vi "Temperature sensors calibration.vi"() -> ()   [LabVIEW 2021]
uses:
  <instrlib>/Lake Shore 350/Public/Data/Sensor Data (Single Reading).vi
  <vilib>/Utility/file.llb/Write Delimited Spreadsheet (DBL).vi
  <instrlib>/Keithley 2450/Keithley 2450.lvlib
  <instrlib>/Lake Shore 350/Lake Shore 350.lvlib
panel:
  out "Chart":T1(graph)
  out "Channel C (Ohm)":dbl format="%#.5f"
  out "Channel B (K)":dbl format="%#.5f"
  out "Channel B (Ohm)":dbl format="%#.5f"
  out "error out write file":errorcluster
  in  "SM1":string
  in  "SM2":string
  out "All data":dbl[][](array[numeric])
  out "SM2 (Omh)":dbl
  in  "error in (no error) 2":errorcluster
  in  "Keithley 2":refnum<visa-resource-name>
  out "VTI Temperature (K)":dbl format="%#.5f"
  out "Waveform Chart":cluster{"Sensor Data":dbl, "Sensor Data":dbl}(graph)
  out "error out":errorcluster
  out "XY Graph":cluster{dbl[], dbl[]}[](graph)
  out "Channel D (Ohm)":dbl format="%#.5f"
  in  "LakeShore 350":refnum<visa-resource-name>="COM4"
  in  "start":bool
  in  "milliseconds to wait":u32=2000
  in  "error in (no error)":errorcluster
  out "SM1 (Omh)":dbl
  in  "Keithley 1":refnum<visa-resource-name>
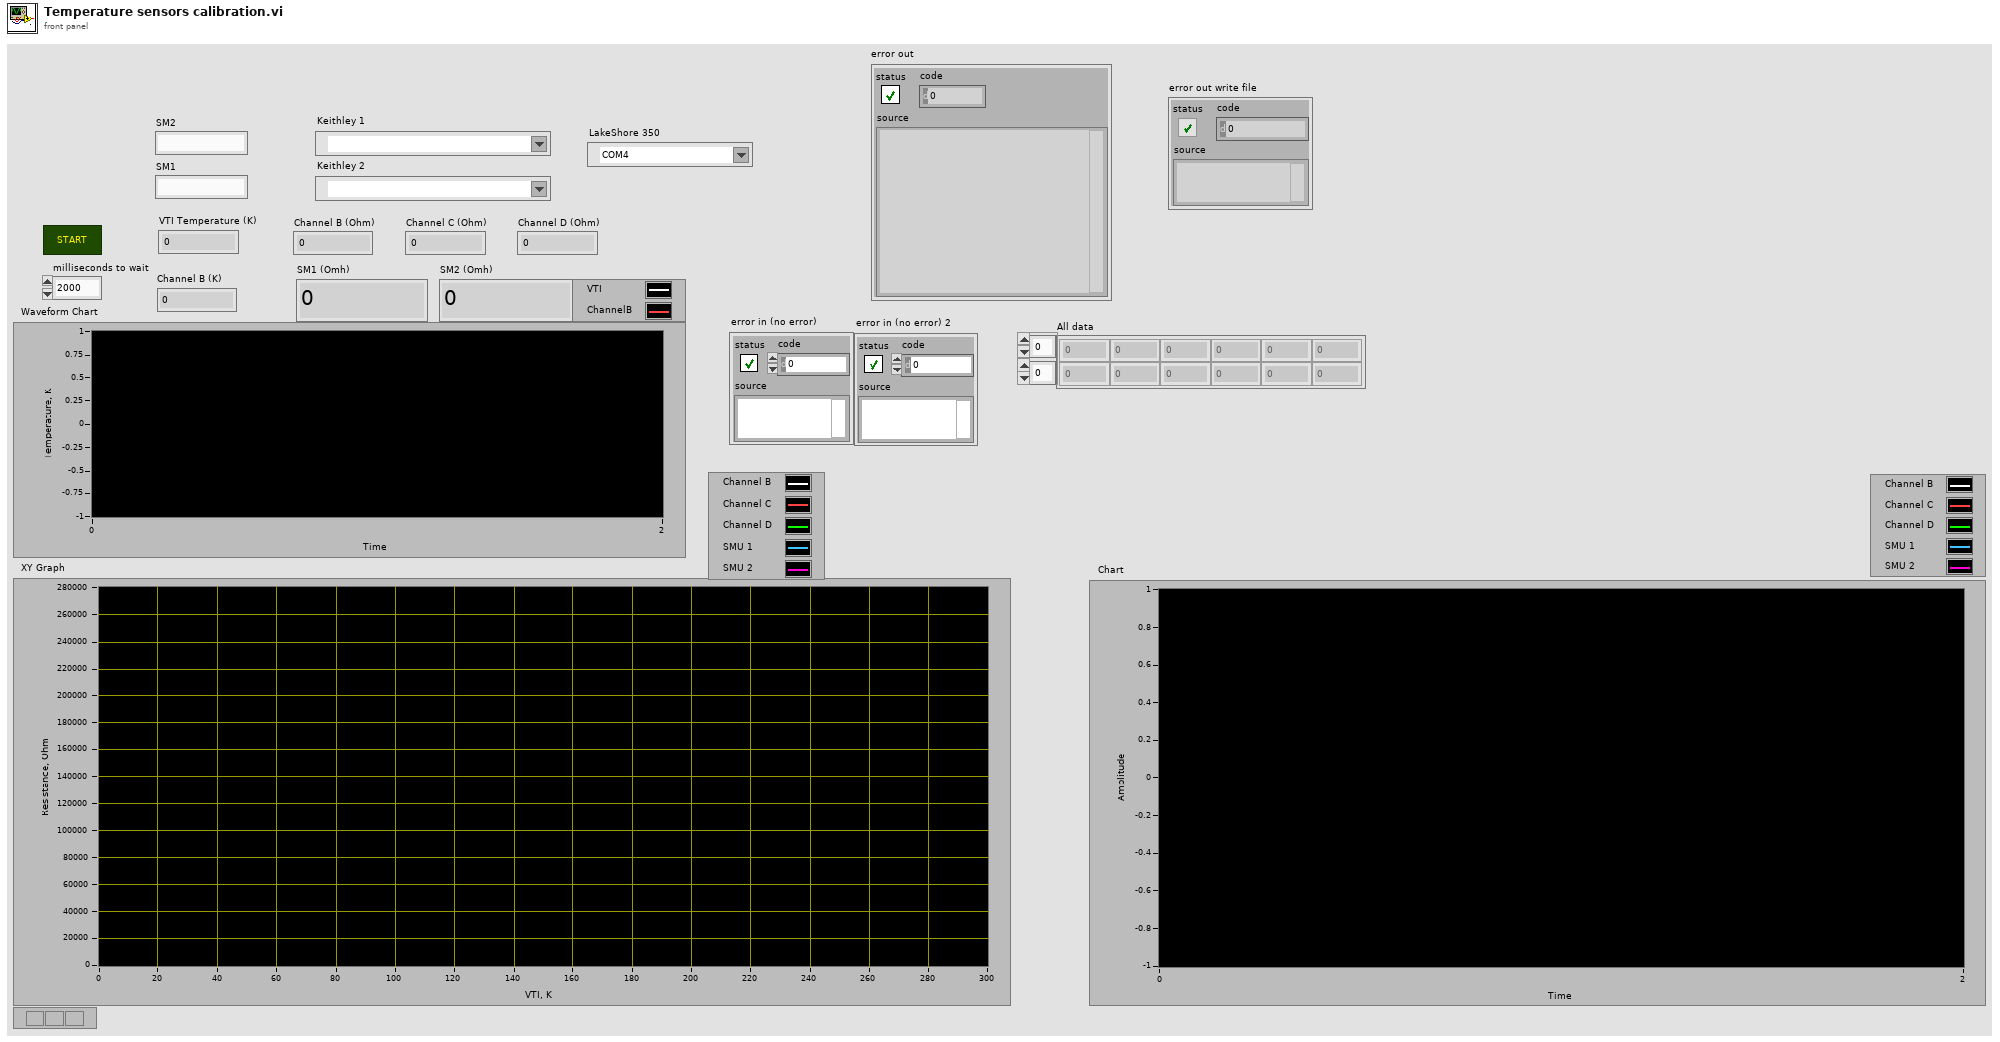
[diagram p1: front panel]
types:
  T1 = cluster{"Sensor Data":dbl, "Sensor Data":dbl, "Sensor Data":dbl, dbl, dbl}
  T2 = enum16{"open", "replace", "create", "open or create", "replace or create", "replace or create with confirmation"}
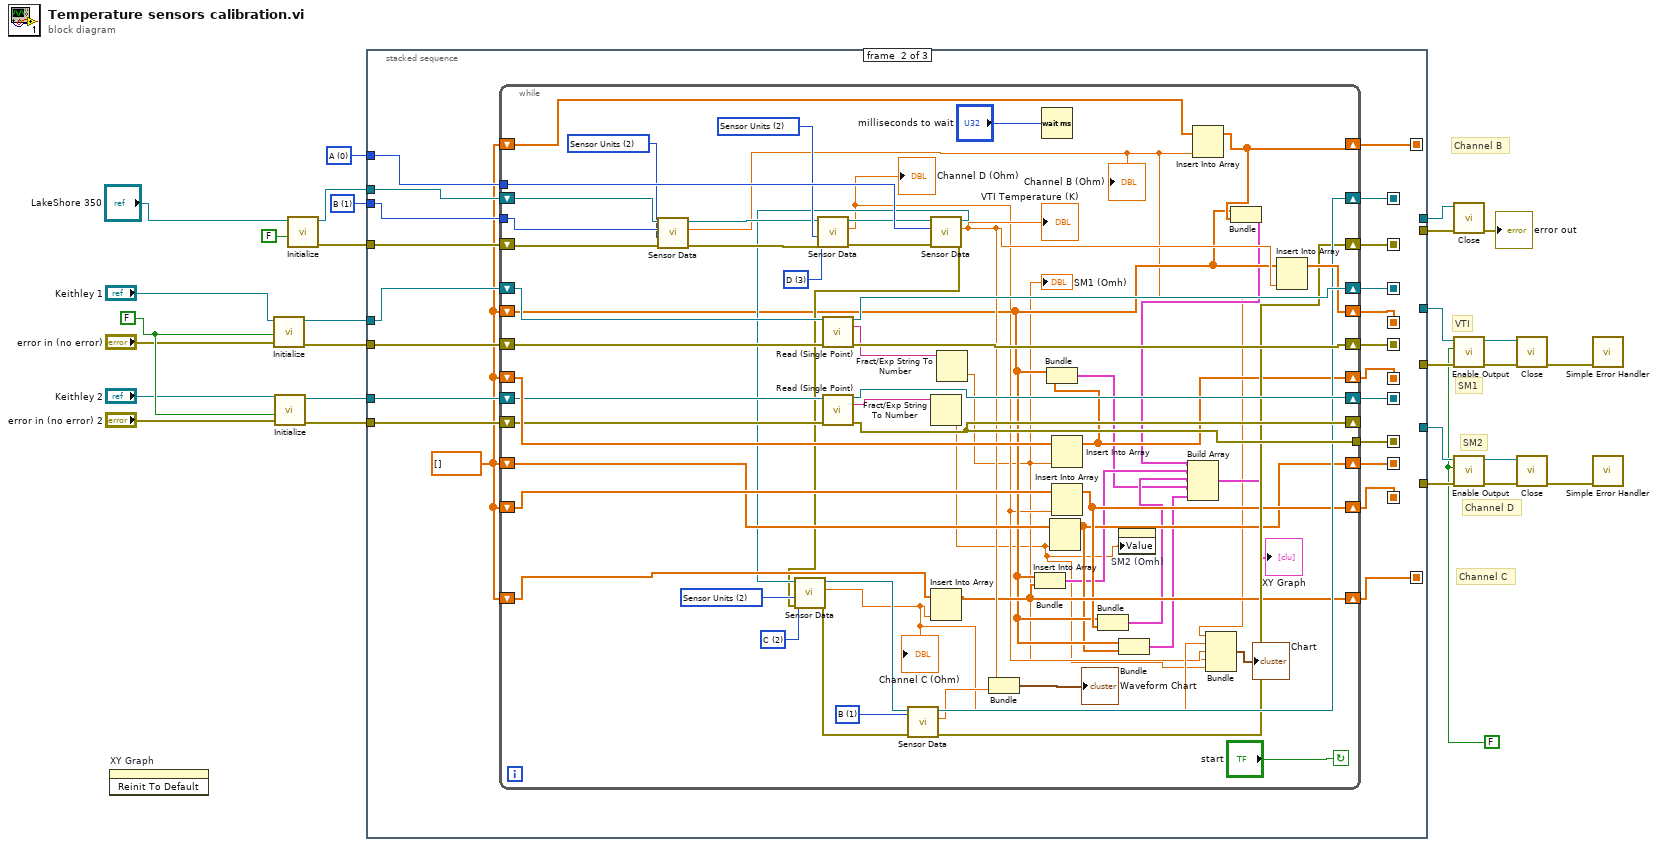
[diagram p0: block diagram]
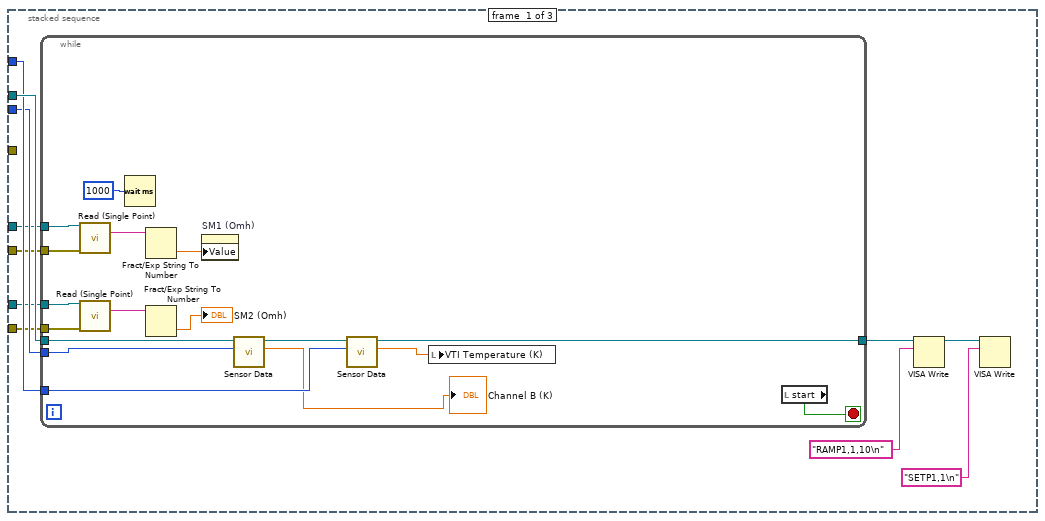
[diagram p2: hidden frame]
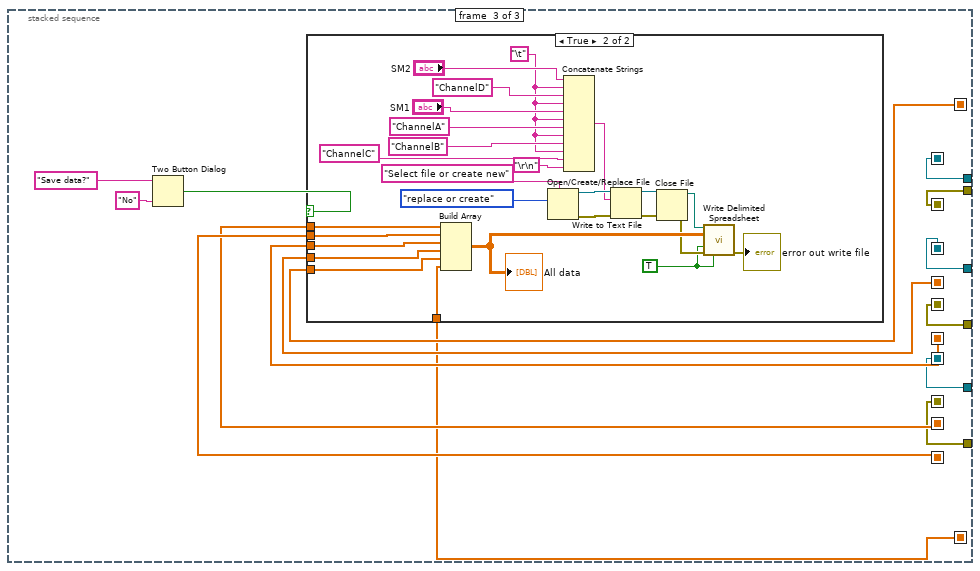
[diagram p3: hidden frame]
diagram:
  w6 = FALSE ("Reset (True)")
  w17 = u16 0 items=["A", "B", "C", "D", "D2", "D3", "D4", "D5"] ("Input (0:A)")
  w21 = u16 1 items=["A", "B", "C", "D", "D2", "D3", "D4", "D5"] ("Input (0:A)")
  w10 = FALSE ("Enable Output (T: Enable)")
  # "Channel C"
  # "Channel B"
  # "Channel D"
  # "SM2"
  # "SM1"
  # "VTI"
  n1 = invoke on="XY Graph" class="XYGraph (strict)" method="Reinit To Default"() -> ()  [unwired: 3 in, 3 out]
  n2 = call <instrlib>:"Initialize.vi"("error in (no error)"="error in (no error)", "Reset (True)"=w6, "VISA resource name"="Keithley 1") -> ("error out"=w15:errorcluster, "VISA resource name out"=w16:refnum<visa-resource-name>)  [unwired: 7 in]
  n3 = call <instrlib>:"Initialize.vi"("error in (no error)"="error in (no error) 2", "Reset (True)"=w6, "VISA resource name"="Keithley 2") -> ("error out"=w14:errorcluster, "VISA resource name out"=w13:refnum<visa-resource-name>)  [unwired: 7 in]
  n4 = call <instrlib>:"Initialize.vi"("Reset (True)"=FALSE, "VISA resource name"="LakeShore 350") -> ("error out"=w22:errorcluster, "VISA resource name out"=w23:refnum<visa-resource-name>)  [unwired: 8 in]
  n5 = stacked-sequence {
    seq-local: [_ w62 _] -> [_ _ w144]
    seq-local: [_ w76 _] -> [_ _ w150]
    seq-local: [_ w75 _] -> [_ _ w149]
    seq-local: [_ w73 _] -> [_ _ w147]
    seq-local: [_ w72 _] -> [_ _ w146]
    seq-local: [_ w63 _] -> [_ _ w145]
    seq-local: [_ w61 _] -> [_ _ w143]
    seq-local: [_ w66 _] -> [_ _ w142]
    seq-local: [_ w64 _] -> [_ _ w141]
    seq-local: [_ w65 _] -> [_ _ w140]
    seq-local: [_ w60 _] -> [_ _ w139]
    seq-local: [_ w58 _] -> [_ _ w138]
    tunnel: w15 -> [w32 w78 _]
    tunnel: w16 -> [w33 w77 _]
    tunnel: [_ _ w150] -> w25
    tunnel: [_ _ w149] -> w26
    tunnel: w23 -> [w40 w71 _]
    tunnel: w22 -> [_ w70 _]
    tunnel: w21 -> [w34 w74 _]
    tunnel: [_ _ w147] -> w20
    tunnel: [_ _ w146] -> w19
    tunnel: w17 -> [w35 w69 _]
    tunnel: w14 -> [w30 w68 _]
    tunnel: w13 -> [w31 w67 _]
    tunnel: [_ _ w141] -> w11
    tunnel: [_ _ w140] -> w12
    frame #0 {
      n6 = while {
        tunnel: w40 -> [w55]
        tunnel: [w53] -> w39
        tunnel: w35 -> [w51]
        tunnel: w34 -> [w50]
        tunnel: w33 -> [w49]
        tunnel: w32 -> [w48]
        tunnel: w31 -> [w44]
        tunnel: w30 -> [w43]
        stop <- w57 stop-if-true
        n7 = call <instrlib>:"Read (Single Point).vi"("VISA resource name"=w49, "error in (no error)"=w48) -> ("Data out"=w47:string)  [unwired: 11 in, 2 out]
        n8 = call <instrlib>:"Read (Single Point).vi"("VISA resource name"=w44, "error in (no error)"=w43) -> ("Data out"=w45:string)  [unwired: 11 in, 2 out]
        n9 = Wait (ms)(milliseconds to wait=u32 1000) -> ()  [unwired: 1 out]
        n10 = Fract/Exp String To Number(string=w47) -> (number=w46:dbl)  [unwired: 3 in, 1 out]
        n11 = Fract/Exp String To Number(string=w45) -> (number=→"SM2 (Omh)":dbl)  [unwired: 3 in, 1 out]
        n12 = property on="SM1 (Omh)" class="DigNum (strict)"("Value"=w46) -> ()  [unwired: 2 in, 2 out]
        n13 = call-poly <instrlib>:"Sensor Data.vi"("Input (0:A)"=w50, "VISA resource name"=w55) -> ("Sensor Data"=→"Channel B (K)":dbl, "VISA resource name out"=w54:refnum<visa-resource-name>)  [unwired: 7 in, 1 out]
        n14 = call-poly <instrlib>:"Sensor Data.vi"("Input (0:A)"=w51, "VISA resource name"=w54) -> ("Sensor Data"=w52:dbl, "VISA resource name out"=w53:refnum<visa-resource-name>)  [unwired: 7 in, 1 out]
        n15 = local write "VTI Temperature (K)"(w52) -> ()
        n16 = local read "start"() -> (w57:bool)
      }
      n17 = VISA Write(VISA resource name=w39, write buffer="RAMP1,1,10\n") -> (VISA resource name out=w37:refnum<visa-resource-name>)  [unwired: 1 in, 2 out]
      n18 = VISA Write(VISA resource name=w37, write buffer="SETP1,1\n") -> ()  [unwired: 1 in, 3 out]
    }
    frame #1 {
      w59 = dbl[] []
      n19 = while {
        shift-right: [w136] -> w75
        shift-left: w78 -> [w131]
        shift-right: [w137] -> w76
        shift-left: w77 -> [w132]
        tunnel: w74 -> [w113]
        shift-right: [w102] -> w73
        shift-left: w71 -> [w116]
        shift-right: [w101] -> w72
        shift-left: w70 -> [w114]
        shift-right: [w96] -> w62
        shift-left: w59 -> [w130]
        shift-right: [w93] -> w63
        shift-left: w59 -> [w129]
        tunnel: w69 -> [w128]
        shift-right: [w125] -> w61
        shift-left: w59 -> [w92]
        shift-right: [w91] -> w66
        shift-left: w59 -> [w118]
        shift-right: [w119] -> _
        shift-left: w68 -> [w122]
        shift-right: [w120] -> w65
        shift-left: w67 -> [w121]
        tunnel: [w119] -> w64
        shift-right: [w95] -> w60
        shift-left: w59 -> [w111]
        shift-right: [w94] -> w58
        shift-left: w59 -> [w109]
        stop <- "start" continue-if-true
        w100 = u16 1 items=["A", "B", "C", "D", "D2", "D3", "D4", "D5"] ("Input (0:A)")
        w107 = u16 2 items=["Kelvin", "Celsius", "Sensor Units"] ("Data Source (0:Kelvin)")
        w108 = u16 2 items=["A", "B", "C", "D", "D2", "D3", "D4", "D5"] ("Input (0:A)")
        w110 = u16 3 items=["A", "B", "C", "D", "D2", "D3", "D4", "D5"] ("Input (0:A)")
        w112 = u16 2 items=["Kelvin", "Celsius", "Sensor Units"] ("Data Source (0:Kelvin)")
        w124 = u16 2 items=["Kelvin", "Celsius", "Sensor Units"] ("Data Source (0:Kelvin)")
        n20 = call-poly <instrlib>:"Sensor Data.vi"("error in (no error)"=w114, "Data Source (0:Kelvin)"=w112, "Input (0:A)"=w113, "VISA resource name"=w116) -> ("error out"=w115:errorcluster, "Sensor Data"=w84:dbl, "VISA resource name out"=w117:refnum<visa-resource-name>)  [unwired: 5 in]
        "Channel B (Ohm)" <- w84
        n21 = call-poly <instrlib>:"Sensor Data.vi"("error in (no error)"=w115, "Data Source (0:Kelvin)"=w124, "Input (0:A)"=w110, "VISA resource name"=w117) -> ("error out"=w126:errorcluster, "Sensor Data"=w82:dbl, "VISA resource name out"=w127:refnum<visa-resource-name>)  [unwired: 5 in]
        "Channel D (Ohm)" <- w82
        n22 = call <instrlib>:"Read (Single Point).vi"("VISA resource name"=w132, "error in (no error)"=w131) -> ("VISA resource name out"=w137:refnum<visa-resource-name>, "Data out"=w135:string, "error out"=w136:errorcluster)  [unwired: 11 in]
        n23 = call <instrlib>:"Read (Single Point).vi"("VISA resource name"=w121, "error in (no error)"=w122) -> ("VISA resource name out"=w120:refnum<visa-resource-name>, "Data out"=w123:string, "error out"=w119:errorcluster)  [unwired: 11 in]
        n24 = call-poly <instrlib>:"Sensor Data.vi"("error in (no error)"=w126, "Input (0:A)"=w128, "VISA resource name"=w127) -> ("error out"=w105:errorcluster, "Sensor Data"=w98:dbl, "VISA resource name out"=w106:refnum<visa-resource-name>)  [unwired: 6 in]
        "VTI Temperature (K)" <- w98
        n25 = call-poly <instrlib>:"Sensor Data.vi"("error in (no error)"=w105, "Data Source (0:Kelvin)"=w107, "Input (0:A)"=w108, "VISA resource name"=w106) -> ("error out"=w103:errorcluster, "Sensor Data"=w83:dbl, "VISA resource name out"=w104:refnum<visa-resource-name>)  [unwired: 5 in]
        "Channel C (Ohm)" <- w83
        n26 = call-poly <instrlib>:"Sensor Data.vi"("error in (no error)"=w103, "Input (0:A)"=w100, "VISA resource name"=w104) -> ("error out"=w101:errorcluster, "Sensor Data"=w99:dbl, "VISA resource name out"=w102:refnum<visa-resource-name>)  [unwired: 6 in]
        n27 = Fract/Exp String To Number(string=w123) -> (number=w80:dbl)  [unwired: 3 in, 1 out]
        n28 = Insert Into Array(array=w109, new element=w83) -> (w94:dbl[])  [unwired: 1 in]
        n29 = Fract/Exp String To Number(string=w135) -> (number=w81:dbl)  [unwired: 3 in, 1 out]
        "SM1 (Omh)" <- w81
        n30 = Bundle("Sensor Data"=w98, "Sensor Data"=w99) -> (→"Waveform Chart":cluster{"Sensor Data":dbl, "Sensor Data":dbl})  [unwired: 1 in]
        n31 = Bundle(w92, w94) -> (w89:cluster{dbl[], dbl[]})  [unwired: 1 in]
        n32 = Wait (ms)(milliseconds to wait="milliseconds to wait") -> ()  [unwired: 1 out]
        n33 = Insert Into Array(array=w118, new element=w80) -> (w91:dbl[])  [unwired: 1 in]
        n34 = Insert Into Array(array=w130, new element=w81) -> (w96:dbl[])  [unwired: 1 in]
        n35 = Bundle(w92, w96) -> (w87:cluster{dbl[], dbl[]})  [unwired: 1 in]
        n36 = Insert Into Array(array=w129, new element=w82) -> (w93:dbl[])  [unwired: 1 in]
        n37 = Bundle(w92, w93) -> (w88:cluster{dbl[], dbl[]})  [unwired: 1 in]
        n38 = property on="SM2 (Omh)" class="DigNum (strict)"("Value"=w80) -> ()  [unwired: 2 in, 2 out]
        n39 = Bundle(w92, w91) -> (w86:cluster{dbl[], dbl[]})  [unwired: 1 in]
        n40 = Insert Into Array(array=w111, new element=w84) -> (w95:dbl[])  [unwired: 1 in]
        n41 = Bundle("Sensor Data"=w84, "Sensor Data"=w83, "Sensor Data"=w82, w81, w80) -> (→"Chart":T1)  [unwired: 1 in]
        n42 = Bundle(w92, w95) -> (w90:cluster{dbl[], dbl[]})  [unwired: 1 in]
        n43 = Build Array(w90, w89, w88, w87, w86) -> (→"XY Graph":cluster{dbl[], dbl[]}[])
        n44 = Insert Into Array(array=w92, new element=w98) -> (w125:dbl[])  [unwired: 1 in]
      }
    }
    frame #2 {
      n45 = Two Button Dialog(message="Save data?", 1:"No" ("F button name (\"Cancel\")")) -> (T button?=w151:bool)  [unwired: 1 in]
      n46 = case shown="True" w151 {
        tunnel: w145 -> [_ w174]
        tunnel: w144 -> [_ w178]
        tunnel: w143 -> [_ w176]
        tunnel: w142 -> [_ w175]
        tunnel: w139 -> [_ w157]
        tunnel: w138 -> [_ w156]
        frame False {
        }
        frame True {
          w154 = "\t"
          w158 = TRUE ("transpose? (no:F)")
          n47 = Build Array(w175, w174, w178, w176, w157, w156) -> (w177:dbl[][])
          "All data" <- w177
          n48 = Open/Create/Replace File(prompt="Select file or create new", operation (0:open)=T2."replace or create") -> (refnum out=w170:refnum<file>, error out=w171:errorcluster)  [unwired: 4 in, 1 out]
          n49 = Concatenate Strings("SM2", w154, "ChannelD", w154, "SM1", w154, "ChannelA", w154, "ChannelB", w154, "ChannelC" ("string"), "\r\n") -> (w167:string)
          n50 = Write to Text File(file (use dialog)=w170, text=w167, error in=w171) -> (refnum out=w168:refnum<file>, error out=w169:errorcluster)  [unwired: 1 in, 1 out]
          n51 = Close File(refnum=w168, error in=w169) -> (path=w161:path, error out=w160:errorcluster)
          n52 = call-poly <vilib>:"Write Delimited Spreadsheet.vi"("file path (dialog if empty)"=w161, "2D data"=w177, "append to file? (new file:F)"=w158, "error in (no error)"=w160, "transpose? (no:F)"=w158) -> ("error out"=→"error out write file":errorcluster)  [unwired: 9 in, 1 out]
        }
      }
    }
  }
  n53 = call <instrlib>:"Close.vi"("error in (no error)"=w19, "VISA resource name"=w20) -> ("error out"=→"error out":errorcluster)  [unwired: 9 in]
  n54 = call <instrlib>:"Enable Output.vi"("error in (no error)"=w26, "Enable Output (T: Enable)"=w10, "VISA resource name"=w25) -> ("error out"=w27:errorcluster, "VISA resource name out"=w28:refnum<visa-resource-name>)  [unwired: 7 in]
  n55 = call <instrlib>:"Enable Output.vi"("error in (no error)"=w11, "Enable Output (T: Enable)"=w10, "VISA resource name"=w12) -> ("error out"=w8:errorcluster, "VISA resource name out"=w9:refnum<visa-resource-name>)  [unwired: 7 in]
  n56 = call <instrlib>:"Close.vi"("error in (no error)"=w27, "VISA resource name"=w28) -> ("error out"=w29:errorcluster)  [unwired: 9 in]
  n57 = call <instrlib>:"Close.vi"("error in (no error)"=w8, "VISA resource name"=w9) -> ("error out"=w7:errorcluster)  [unwired: 9 in]
  n58 = call <vilib>:"Simple Error Handler.vi"("error in (no error)"=w29) -> ()  [unwired: 4 in, 5 out]
  n59 = call <vilib>:"Simple Error Handler.vi"("error in (no error)"=w7) -> ()  [unwired: 4 in, 5 out]
